vi "Keithley_Iterator.vi"(0 "VISA resource name":refnum<visa-resource-name>, 1 "High Voltage":dbl, 2 "Low Voltage":dbl, 3 "Initial Voltage":dbl, 5 "Iteration Input":i32, 7 "Current Voltage":dbl, 11 "error in (no error)":errorcluster, 12 "Voltage Step":dbl, 13 "Compliance  Level (0.1)":dbl=0.1) -> (4 "VISA resource name out":refnum<visa-resource-name>, 6 "Iteration Output":i32, 8 "New Voltage":dbl, 10 "END?":bool, 15 "error out":errorcluster)   [LabVIEW 2021]
uses:
  <instrlib>/Keithley 24XX/Keithley 24XX.lvlib
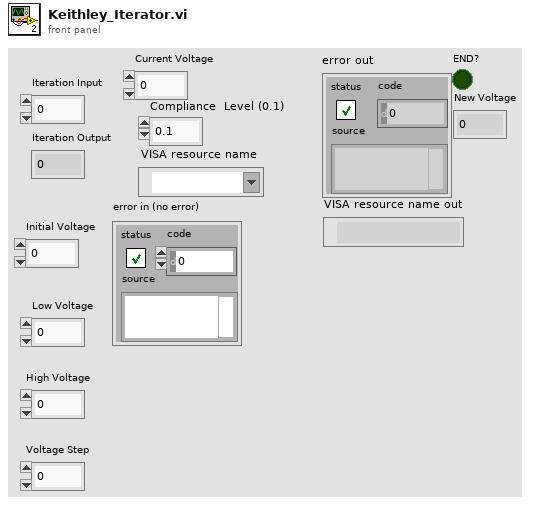
[diagram p1: front panel]
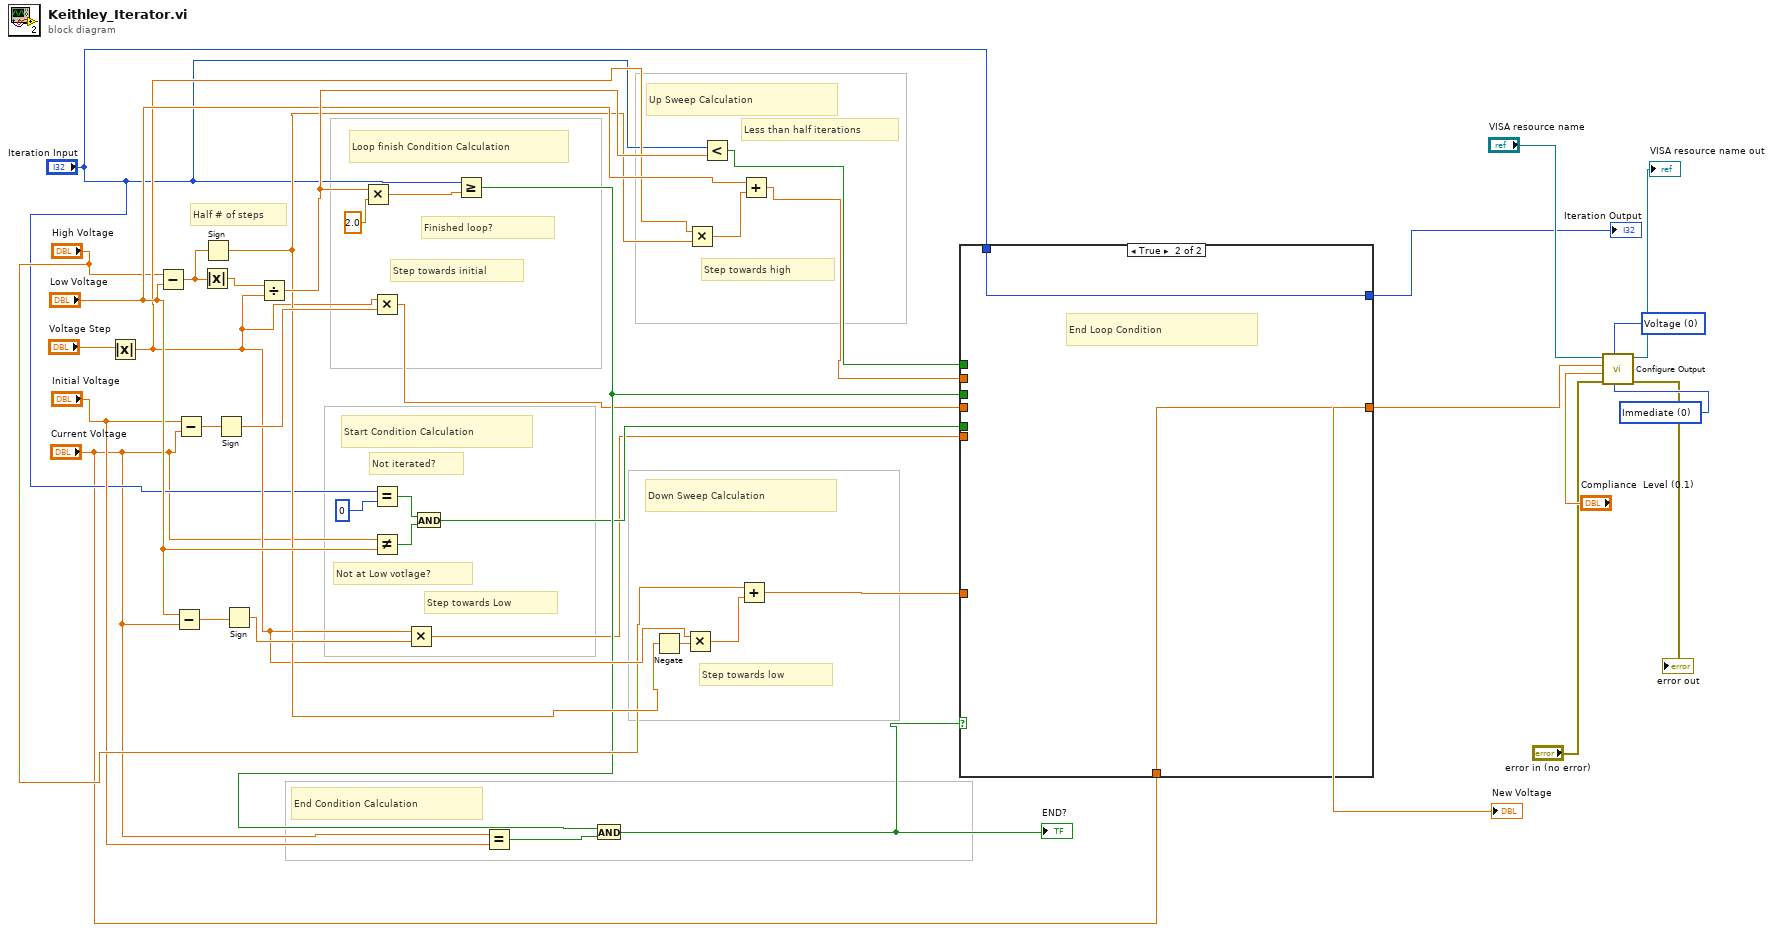
[diagram p0: block diagram]
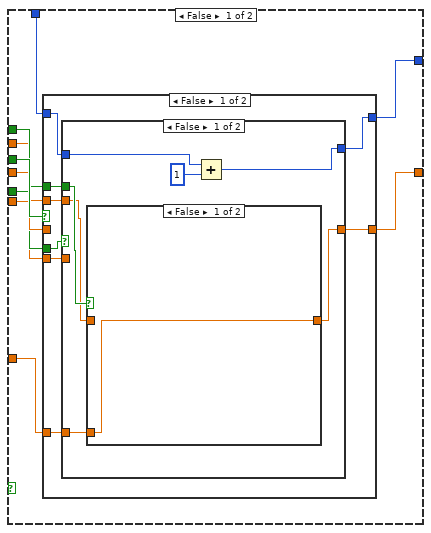
[diagram p2: hidden frame]
diagram:
  w40 = u16 0 items=["Immediate", "Triggered"] ("Output Type  (0: Immediate)")
  w41 = u16 0 items=["Voltage", "Current"] ("Source Mode  (0: Voltage)")
  # "End Condition Calculation"
  # "Step towards low"
  # "Less than half iterations"
  # "Step towards high"
  # "Step towards Low"
  # "Not at Low votlage?"
  # "Not iterated?"
  # "Finished loop?"
  # "Step towards initial"
  # "Half # of steps"
  # "Down Sweep Calculation"
  # "Up Sweep Calculation"
  # "Start Condition Calculation"
  # "Loop finish Condition Calculation"
  n1 = Absolute Value(x="Voltage Step") -> (abs(x)=w20:dbl)
  n2 = Subtract(x="High Voltage", y="Low Voltage") -> (x-y=w25:dbl)
  n3 = Subtract(x="Low Voltage", y="Current Voltage") -> (x-y=w29:dbl)
  n4 = Subtract(x="Initial Voltage", y="Current Voltage") -> (x-y=w34:dbl)
  n5 = Absolute Value(x=w25) -> (abs(x)=w37:dbl)
  n6 = Sign(1:w25) -> (0:w21:dbl)
  n7 = Sign(1:w34) -> (0:w33:dbl)
  n8 = Sign(1:w29) -> (0:w28:dbl)
  n9 = Divide(x=w37, y=w20) -> (x/y=w27:dbl)
  n10 = Multiply(x=w27, y=2.0) -> (x*y=w35:dbl)
  n11 = Multiply(x=w20, y=w33) -> (x*y=w10:dbl)
  n12 = Equal?(x="Iteration Input", y=0) -> (x = y?=w30:bool)
  n13 = Not Equal?(x="Current Voltage", y="Low Voltage") -> (x != y?=w31:bool)
  n14 = Multiply(x=w20, y=w28) -> (x*y=w8:dbl)
  n15 = And(x=w30, y=w31) -> (x .and. y?=w9:bool)
  n16 = Greater Or Equal?(x="Iteration Input", y=w35) -> (x >= y?=w11:bool)
  n17 = Equal?(x="Current Voltage", y="Initial Voltage") -> (x = y?=w13:bool)
  n18 = And(x=w11, y=w13) -> (x .and. y?=w12:bool)
  "END?" <- w12
  n19 = Negate(x=w21) -> (-x=w22:dbl)
  n20 = Multiply(x=w20, y=w22) -> (x*y=w23:dbl)
  n21 = Multiply(x=w20, y=w21) -> (x*y=w24:dbl)
  n22 = Less?(x="Iteration Input", y=w27) -> (x < y?=w6:bool)
  n23 = Add(x="High Voltage", y=w23) -> (x+y=w4:dbl)
  n24 = Add(x="Low Voltage", y=w24) -> (x+y=w5:dbl)
  n25 = case shown="True" w12 {
    tunnel: w11 -> [w51 _]
    tunnel: w10 -> [w50 _]
    tunnel: w9 -> [w49 _]
    tunnel: w8 -> [w48 _]
    tunnel: "Iteration Input" -> [w47 w74]
    tunnel: w6 -> [w46 _]
    tunnel: w5 -> [w45 _]
    tunnel: w4 -> [w44 _]
    tunnel: [w43 w73] -> w3
    tunnel: [w42 w74] -> w2
    tunnel: "Current Voltage" -> [_ w73]
    frame False {
      n26 = case shown="False" w51 {
        tunnel: w50 -> [_ w72]
        tunnel: [w57 w72] -> w43
        tunnel: w49 -> [w59 _]
        tunnel: w48 -> [w58 _]
        tunnel: w47 -> [w56 w71]
        tunnel: [w55 w71] -> w42
        tunnel: w46 -> [w54 _]
        tunnel: w45 -> [w53 _]
        tunnel: w44 -> [w52 _]
        frame False {
          n27 = case shown="False" w59 {
            tunnel: w58 -> [_ w70]
            tunnel: [w61 w70] -> w57
            tunnel: w56 -> [w65 w69]
            tunnel: [w64 w69] -> w55
            tunnel: w54 -> [w63 _]
            tunnel: w53 -> [w62 _]
            tunnel: w52 -> [w60 _]
            frame False {
              n28 = case shown="False" w63 {
                tunnel: [w67 w68] -> w61
                tunnel: w62 -> [_ w68]
                tunnel: w60 -> [w67 _]
                frame False {
                }
                frame True {
                  # "Upsweep condition"
                }
              }
              n29 = Add(x=w65, y=1) -> (x+y=w64:i32)
            }
            frame True {
              # "Haven't started program, step towards LOW condition."
            }
          }
        }
        frame True {
          # "Finished prog, step towards initial condition."
        }
      }
    }
    frame True {
      # "End Loop Condition"
    }
  }
  "Iteration Output" <- w2
  "New Voltage" <- w3
  n30 = call <instrlib>:"Configure Output.vi"("Output Type  (0: Immediate)"=w40, "Source Mode  (0: Voltage)"=w41, "error in (no error)"="error in (no error)", "Compliance  Level (0.1)"="Compliance  Level (0.1)", "Output Level (0)"=w3, "VISA resource name"="VISA resource name") -> ("error out"=→"error out":errorcluster, "VISA resource name out"=→"VISA resource name out":refnum<visa-resource-name>)  [unwired: 4 in]
